vi "PH_Timing.PC PU GD Info.vi"(0 "i ref in":refnum<vi>, 1 "PU":T1, 2 "GD Instance Name":string, 3 "PU Channel":i32(ring)=4 items=["System (To)", "Channel A", "Channel B", "Channel C", "Channel D", "Channel E", "Channel F", "Channel G", "Channel H"], 5 "error in":errorcluster) -> (14 "i ref out":refnum<vi>, 19 "error out":errorcluster)   [LabVIEW 2014, in "PH_Timing.lvlib"]
doc: "This VI writes the incoming information to own attributes and sets GUI elements."
uses:
  PH_Timing.lvlib
  PH_PP_Common/PH_PP_Common.PUs.ctl
  PH_Common/PH_Common.lvlib
  PH_PP_Common/PH_PP_Common.lvlib
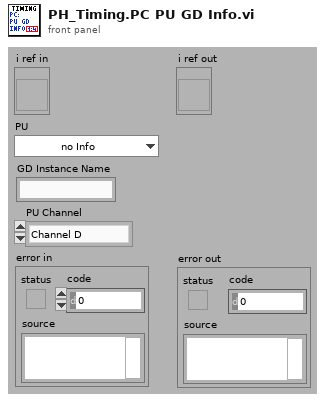
[diagram p1: front panel]
types:
  T1 = typedef "PH_PP_Common.lvlib/PH_PP_Common.PUs.ctl" = enum16{"no Info", "PA-19mm-1", "PA-19mm-2", "PA-45mm-PILC", "PA-45mm-MAIN", "MA-PU-1", "MA-PU-2", "MA-PU-3", "MA-PU-4", "MA-PU-5", "MA-PU-6", "MA-FR", "MA-PILC", "PA-45mm-DP"}
  T2 = typedef "PH_Timing.lvlib/PH_Timing.i attribute.ctl" = cluster{"Sequencer":cluster{"linked?":bool, "Proc State":string, "Ref State":refnum<vi>}, "Gate Generator":cluster{"GD":cluster{"Device Status":T3, "linked?":bool}, "Settings":T4, "GUI Ref":refnum<vi>}, "Interlock Bypass":cluster{"Instancename":string, "Switch linked?":bool, "Device Status":T3, "Ref Status":refnum<vi>}, "Roughtuner":cluster{"Settings":T5, "GUI Ref":refnum<vi>, "GD":cluster{"Device Status":T3, "linked?":bool}}, "0,5Hz Gater":cluster{"Settings":T6, "GUI Ref":refnum<vi>, "GD":cluster{"Device Status":T3, "linked?":bool}}, "Slow Trigger":cluster{"Settings":T7, "GUI Ref":refnum<vi>, "Service ID Delay":i32, "Service ID Ext Trig":i32, "Wanted Settings":T7}, "Timing Mode":cluster{"Mode":T8, "GUI Ref":refnum<vi>, "Service ID T2":i32, "Service ID Mode":i32, "Wanted Mode":T8}, "ns Generator":cluster{"Settings":T9, "ns Generator Settings":refnum<vi>, "GD":cluster{"Device Status":T3, "linked?":bool}}, "Phase FEs":cluster{"Settings":T12, "GUI Ref":refnum<vi>, "Service ID Phase":i32, "Wanted Settings":T12}, "GD GUI Refs":refnum<vi>[], "Heads":T13[], "GUI Ref Delete":refnum<vi>}
  T3 = typedef "PH_StatusHandler.lvlib/PH_StatusHandler.Status.ctl" = i16
  T4 = typedef "PH_Timing.lvlib/PH_Timing.GateGen.ctl" = cluster{"Instance":string, "Channel Gate":i32, "Channel T2":i32, "Width Gate":dbl, "Width T2":dbl, "Delay Gate":dbl, "Delay T2":dbl, "Gate activ":bool, "T2 activ":bool, "System Mode":enum16{"Normal", "Single", "Burst", "Duty Cycle"}}
  T5 = typedef "PH_Timing.lvlib/PH_Timing.Roughtuner.ctl" = cluster{"Instance":string, "Phase PHELIX / UNILAC":cluster{"Channel":u16, "relative to":u16, "Delay [ms]":dbl}, "Pulse Length":cluster{"Channel":u16, "relative to":u16, "Delay [ms]":dbl}, "Trigger":cluster{"externally?":bool, "Rate [Hz]":dbl}}
  T6 = typedef "PH_Timing.lvlib/PH_Timing.0.5HzGater.ctl" = cluster{"Instance":string, "Channel ns FE Delay":i32, "Channel 0.5Hz":i32, "Width ns FE Delay":dbl, "Width 0.5Hz":dbl, "Delay ns FE Delay":dbl, "Delay 0.5Hz":dbl, "ns FE Delay active":bool, "0.5Hz activ":bool, "ns FE Delay inverted":bool, "0.5Hz inverted":bool}
  T7 = typedef "PH_Timing.lvlib/PH_Timing.Slow Trigger Settings.ctl" = cluster{"Delay":dbl, "externally triggered?":bool}
  T8 = typedef "PH_Timing.lvlib/PH_Timing.Timing Mode.ctl" = cluster{"T2":i16, "Modeselector":enum32{"10 Hz", "0.5 Hz", "Shot"}}
  T9 = typedef "PH_Timing.lvlib/PH_Timing.ns Generator.ctl" = cluster{"Instance":string, "Phase fs / ns FE":cluster{"Channel":T10, "Settings":T11}}
  T10 = typedef "Stanford Research DG645 - Driver.lvlib/Channel.ctl" = i32
  T11 = typedef "PH_SRDG645.lvlib/PH_SRDG645.Channel Settings.ctl" = cluster{"Delay [s]":dbl, "relative to":i32}
  T12 = typedef "PH_Timing.lvlib/PH_Timing.Phase FEs.ctl" = cluster{"Phase":dbl}
  T13 = typedef "PH_Timing.lvlib/PH_Timing.PU Data.ctl" = cluster{"linked?":bool, "Data":T14, "GD":cluster{"Device Status":T3, "linked?":bool}, "GUI Ref":refnum<vi>, "PU":T1}
  T14 = typedef "PH_Timing.lvlib/PH_Timing.PU Info.ctl" = cluster{"Act CH?":bool, "GD":string, "CH":i32, "Delay":dbl, "active":bool, "in Use?":bool}
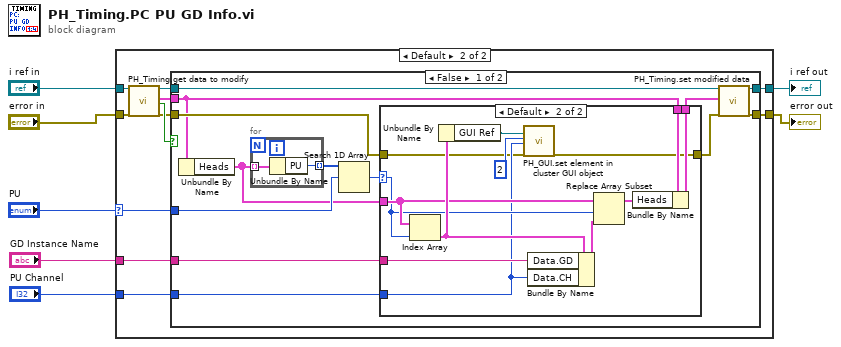
[diagram p0: block diagram]
diagram:
  n1 = case shown="Default" "PU" {
    selector: "PU" -> [_ w10]
    tunnel: [w8 w18] -> w7
    tunnel: "error in" -> [w8 w16]
    tunnel: [w9 w15] -> w5
    tunnel: "i ref in" -> [w9 w13]
    tunnel: "GD Instance Name" -> [_ w12]
    tunnel: "PU Channel" -> [_ w11]
    frame "no Info" {
    }
    frame Default {
      n2 = call "PH_Timing.get data to modify.vi"("i ref in"=w13, "error in (no error)"=w16) -> ("i ref out"=w14:refnum<vi>, "i attribute"=w19:T2, "timed out"=w20:bool, "error out"=w17:errorcluster)  [unwired: 14 in]
      n3 = case shown="False" w20 {
        tunnel: w14 -> [w33 w52]
        tunnel: [w32 w52] -> w15
        tunnel: w17 -> [w30 w51]
        tunnel: [w31 w51] -> w18
        tunnel: w19 -> [w29 _]
        tunnel: w10 -> [w28 _]
        tunnel: w11 -> [w27 _]
        tunnel: w12 -> [w22 _]
        frame False {
          n4 = Unbundle By Name(w29) -> ("Heads"=w21:T13[])
          n5 = for {
            tunnel: w21 -> [w50] mode=indexing
            tunnel: [w49] -> w26 mode=indexing
            n6 = Unbundle By Name(w50) -> ("PU"=w49:T1)
          }
          n7 = Search 1D Array(1D array=w26, element=w28) -> (index of element=w23:i32)  [unwired: 1 in]
          n8 = case shown="Default" w23 {
            selector: w23 -> [_ w43]
            tunnel: w30 -> [w35 w37]
            tunnel: [w35 w41] -> w25
            tunnel: w29 -> [w34 w48]
            tunnel: [w34 w47] -> w24
            tunnel: w21 -> [_ w45]
            tunnel: w22 -> [_ w42]
            tunnel: w27 -> [_ w38]
            frame -1 {
            }
            frame Default {
              n9 = Index Array(array=w45, index=w43) -> (element=w46:T13)
              n10 = Unbundle By Name(w46) -> ("GUI Ref"=w40:refnum<vi>)
              n11 = call "PH_GUI.set element in cluster GUI object.vi"("Cluster Ref"=w40, "Cluster index"=2, "Value"=w38, "error in (no error)"=w37) -> ("error out"=w41:errorcluster)  [unwired: 15 in]
              n12 = Bundle By Name(cluster=w46, "Data.GD"=w42, "Data.CH"=w38) -> (w44:T13)
              n13 = Replace Array Subset(array=w45, new element=w44, index=w43) -> (w36:T13[])
              n14 = Bundle By Name(cluster=w48, "Heads"=w36) -> (w47:T2)
            }
          }
          n15 = call "PH_Timing.set modified data.vi"("i ref in"=w33, "i attribute"=w24, "error in (no error)"=w25) -> ("i ref out"=w32:refnum<vi>, "error out"=w31:errorcluster)  [unwired: 15 in]
        }
        frame True {
        }
      }
    }
  }
  "error out" <- w7
  "i ref out" <- w5
